vi "CPP-BLplotter.vi"(0 "Plot Array":cluster{dbl[], dbl[]}[](array[cluster])=[{[500.0, 500.0, 953.54, 215.0, 270.0, 320.0, 445.0, 525.0, 600.0, 675.0, 750.0, 825.0, 900.0, 960.0, 1010.0, 1060.0], [4.614524, 4.54365, 5.818368, 0.1374656, 0.6662545, 1.465458, 3.619824, 4.848976, 5.887329, 5.940571, 6.152151, 5.717487, 5.600293, 5.40069, 5.154843, 5.121789]}, {[100.0, 150.0, 215.0, 270.0, 320.0, 445.0, 525.0, 600.0, 675.0, 750.0, 825.0, 900.0, 960.0, 1010.0, 1060.0], [0.002314715, -0.00693192, 0.120417, 0.6880509, 1.519176, 3.513709, 5.065183, 6.116033, 6.096773, 5.938465, 5.593788, 5.5597, 5.387002, 5.304077, 4.887903]}] {"?" format="%.2f"; "?" format="%.2f"}, 1 "Job Directory":path=path "/G4_2_HD/Users/paulhayden/Documents/Projects/Westlakes_resolution") -> (2 "Saved Automatically?":bool, 3 "gnuplotScript":string="set term epslatex\nset output \"Plot.eps\"\nset xlabel '$Distance~(m)$'\nset ylabel '$DF~(s/m^3)\\times10^6$'\nset samples 1000\nset pointsize 1.00\nset title '$B38~Centreline~Glc$' 0, 0\nset size 0.75,0.9\n\n#set key 450, -2.5833\n unset key\nset label 1 '~~~~~~~~~~~Angle~(deg)~=~0' at -100, -2.58\nset label 2 '~~~~~~~~~~~Height~(m)~=~5' at -100, -3.27\n set xrange [0 : 500] \n# set autoscale x \n set yrange [0.10000 : 7]\n# set autoscale y \n\nplot \"B38_Centreline_Glc.dat\" index 0 using 1:2 axes x1y1 title '$File=B38R~DDD.xls$' with points 1 1, \\\n\"B38_Centreline_Glc.dat\" index 1 using 1:2 axes x1y1 title '$File=B38R~DDD~1.xls$' with points 1 3", 4 "Plot data file":path)   [LabVIEW 2013]
uses:
  Results_plotter_Global.vi
panel:
  in  "Tab Control":enum32{"Good Shit", "Boring Shit"}(tab)
  in  "HeightJitterFraction":dbl=0.03
  in  "Spectra Files:":path
  out "Spectrum":cluster{dbl[], dbl[]}[](graph)
  in  "Cancel Button":bool
  in  "Print Button":bool
  out "U,L(U)":cluster{dbl[], dbl[]}[](graph)
  out "TI,Sigma":cluster{dbl[], dbl[]}[](graph)
  in  "Use for:":enum16{"\nU", "\nLambda", "\nTI", "\nSigma"}[](array[ring])=[enum."\nU", enum."\nTI", enum."\nSigma", enum."\nLambda"]
  out "Incoming Titles":string[](array[string])
  in  "Plot Title":u16(ring) items=["Title String Only", "Number of Measurements", "Date::", "Profile::", "Multi Run:Start Time:", "Multi Run:Row:Type", "Multi Run:Row:Number", "Point:Time:", "Time:Stamp:", "Measuring:Instrument:Type", "Comments::", "Run:Messages:", "X_{HF}:(mm):", "Y_{HF}:(mm):", "Z_{HF}:(mm):", "X_{5HP}:(mm):", "Y_{5HP}:(mm):", "Z_{5HP}:(mm):", "Repeat::", "U_{HF}/U_{ref}::", "U_{5HP}/U_{ref}::", "U_{HF}/U_{5HP}::", "TI_{HF}:%:", "\\sigma_{HF}/U_{ref}::", "TI_{U(5HP)}:%:", "Vmag_{5HP}/U_{ref}::", "V_{5HP}/U_{5HP}::", "W_{5HP}/U_{5HP}::", "U_{ref}::", "U_{HF}::", "L(U):Est:(m)", "Tau(HF)::", "uhf^2::", "uhf^3/(uhf^2)^1.5::", "(uhf^4/(uhf^2)^2) -3::", "HW (Uhf):Standard Error:in Mean", "HW (Uhf):Standard Error:in Variance", "HW:Cal:", "Vmag_{5HP}::", "U_{5HP}::", "V_{5HP}::", "W_{5HP}::", "Vmag_SD::", "U_SD::", "V_SD::", "W_SD::", "Tau(5HP1)::(nose)", "Tau(5HP2)::(bottom)", "Tau(5HP3)::(top)", "Tau(5HP4)::(side)", "Tau(5HP5)::(side)", "GoodFraction::", "5HP:Mode:", "5HP:ReturnType:", "Reference:Temperature:Used for Corrections", "Atmos:Pressure:Used for Corrections", "Av Analogue:Sampling:Rate", "No of:Analogue:Samples", "No Of:Measurement:Blocks", "Flow:Measurement:Time", "X:(URef):(mm)", "Y:(URef):(mm)", "Z:(URef):(mm)", "Original:Results:Filename", "Current:Data:Filename", "Current:Data File:1st Folder level", "Current:Data File:2nd Folder level", "Current:Data File:3rd Folder level", "Current:Data File:4th Folder level", "Current:File:Number", "Raw:Data:Filename"]
  in  "Filename Max length":i32=255
  out "Final Title":string="B38 Centreline Glc"
  out "Path":path
  in  "Plot Title Post Block":string
  in  "Plot Title Pre Block":string
  in  "Show Script Editor?":bool
  out "t":string
  in  "OpenLogfile?":bool
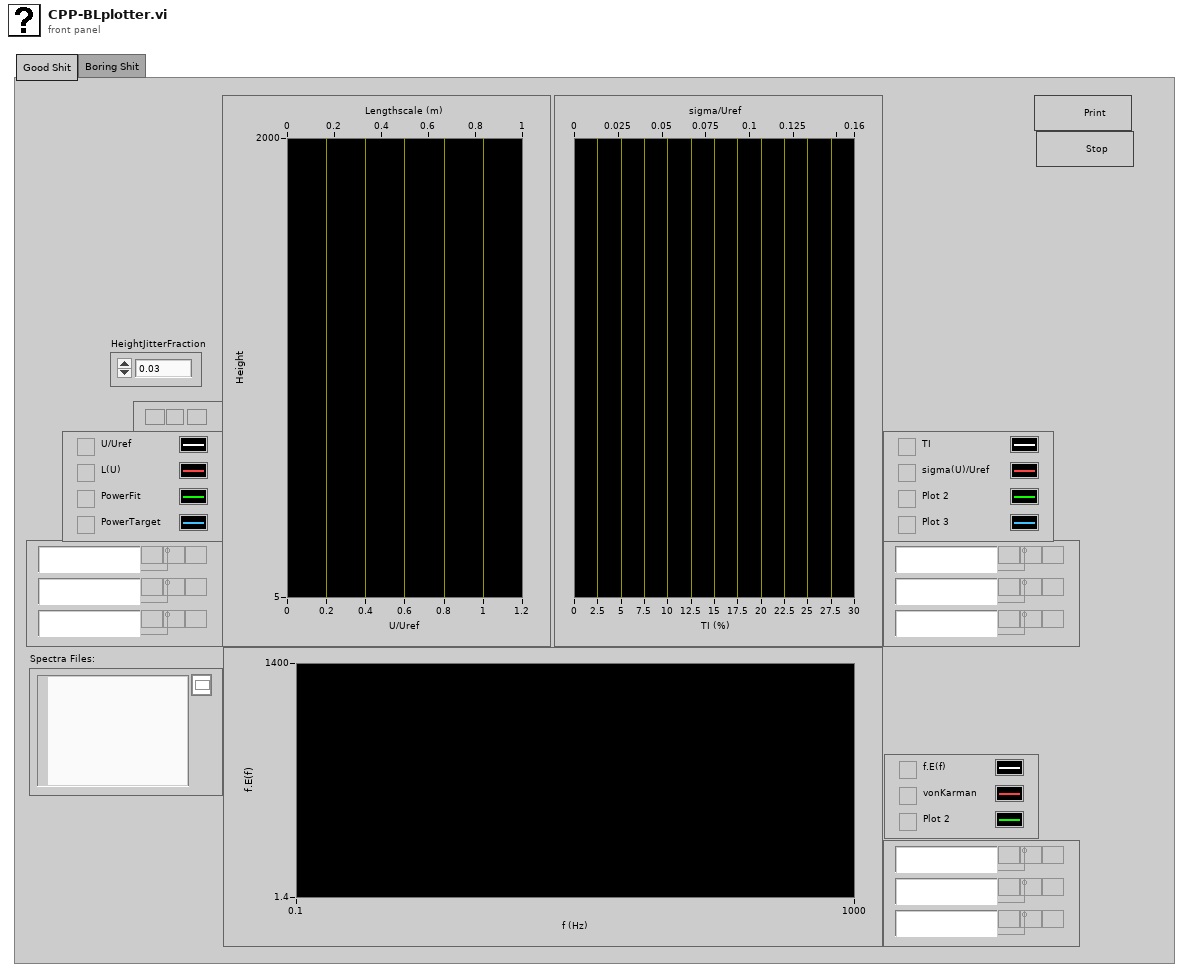
[diagram p1: front panel]
types:
  T1 = typedef "LVRangeTypeDef.ctl" = cluster{"Minimum":dbl, "Maximum":dbl, "Increment":dbl, "Minor Increment":dbl, "Start":dbl}
  T2 = typedef "minAndMax.ctl" = cluster{"Min":T3, "Max":T3}
  T3 = typedef "AutoManualNumber.ctl" = cluster{"Auto":bool, "Value":dbl}
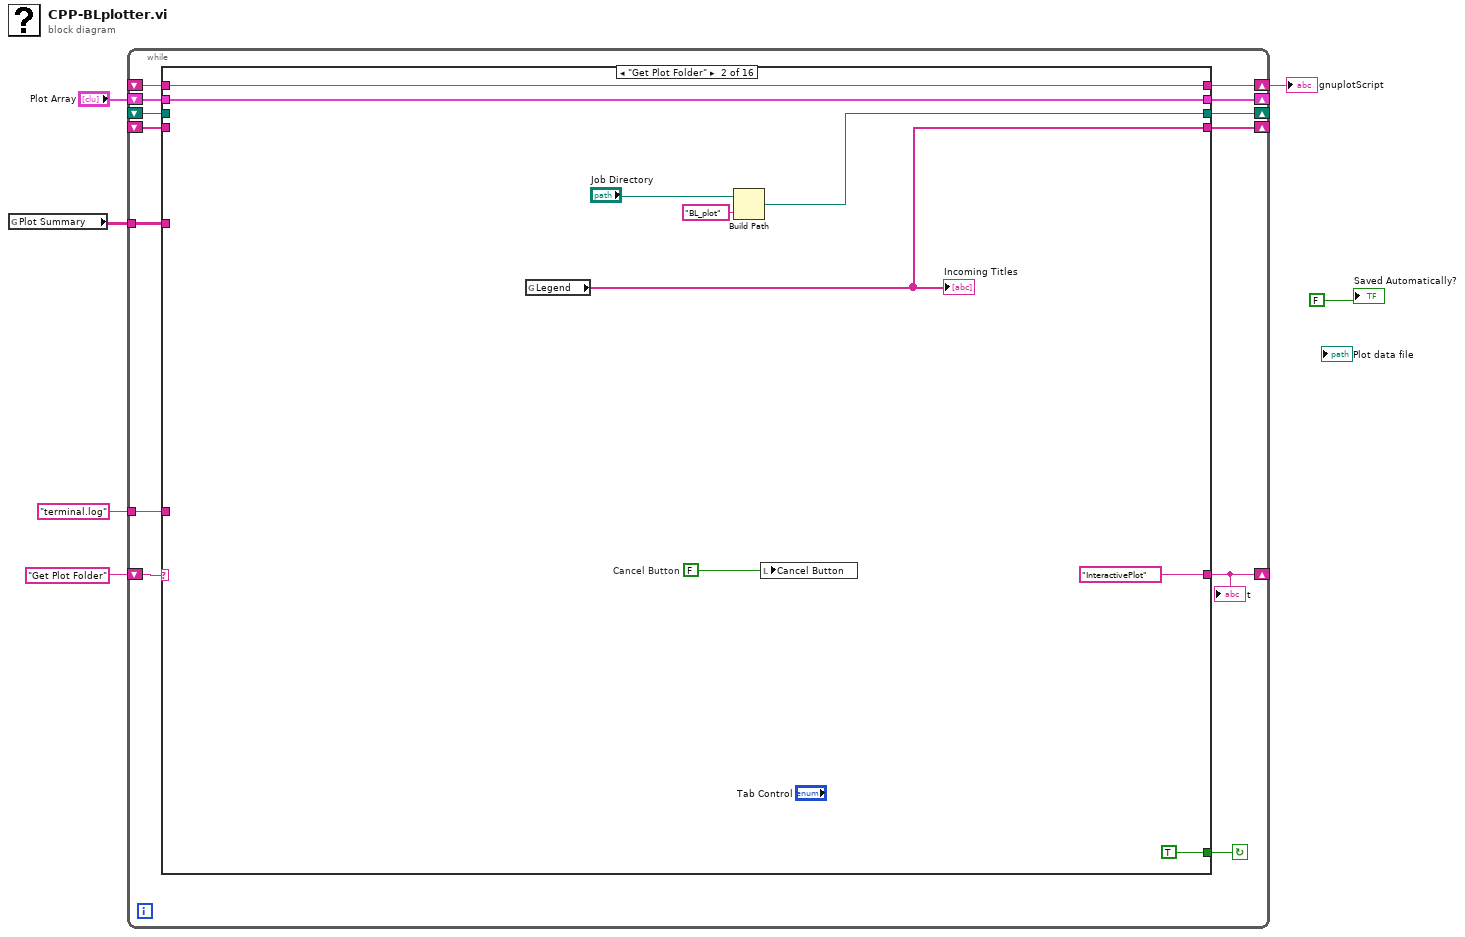
[diagram p0: block diagram]
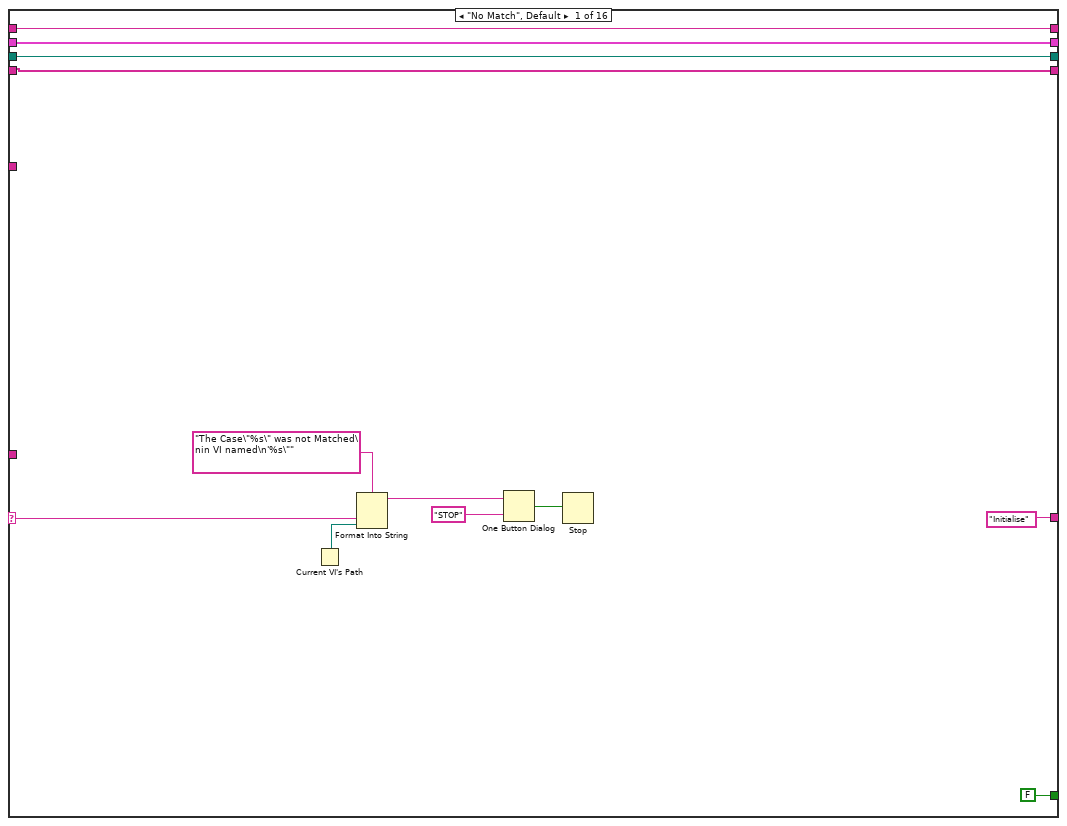
[diagram p2: hidden frame]
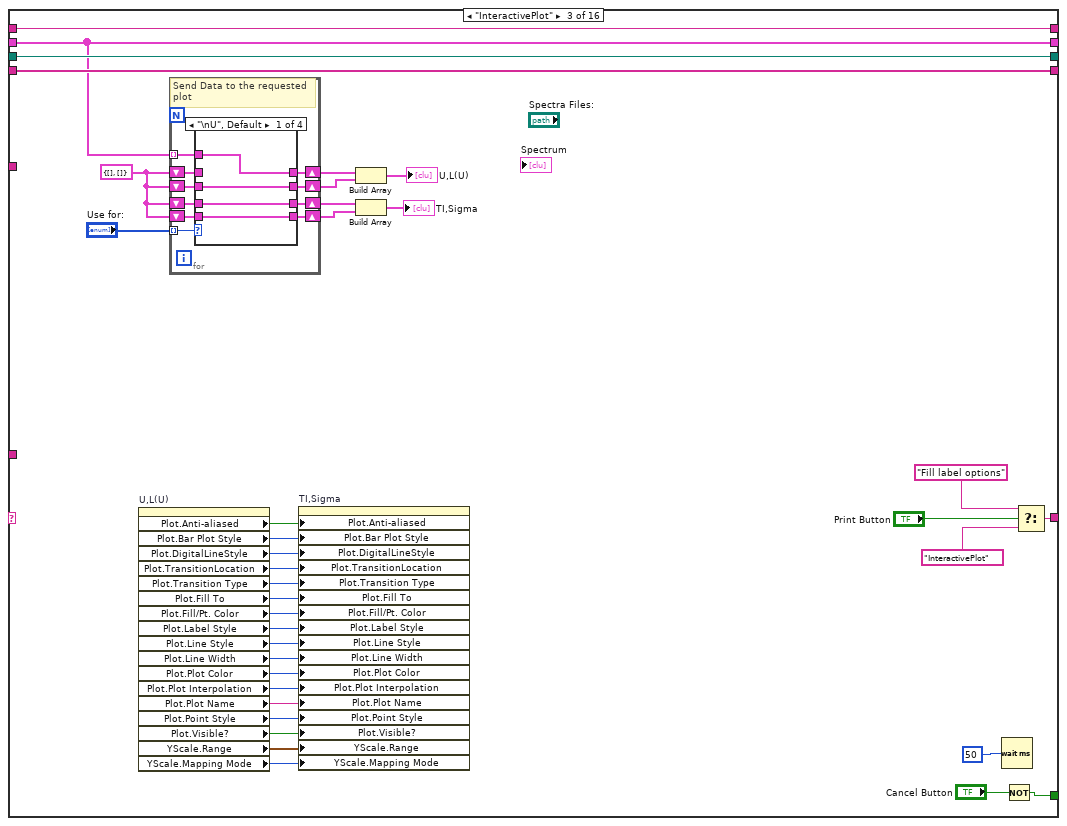
[diagram p3: hidden frame]
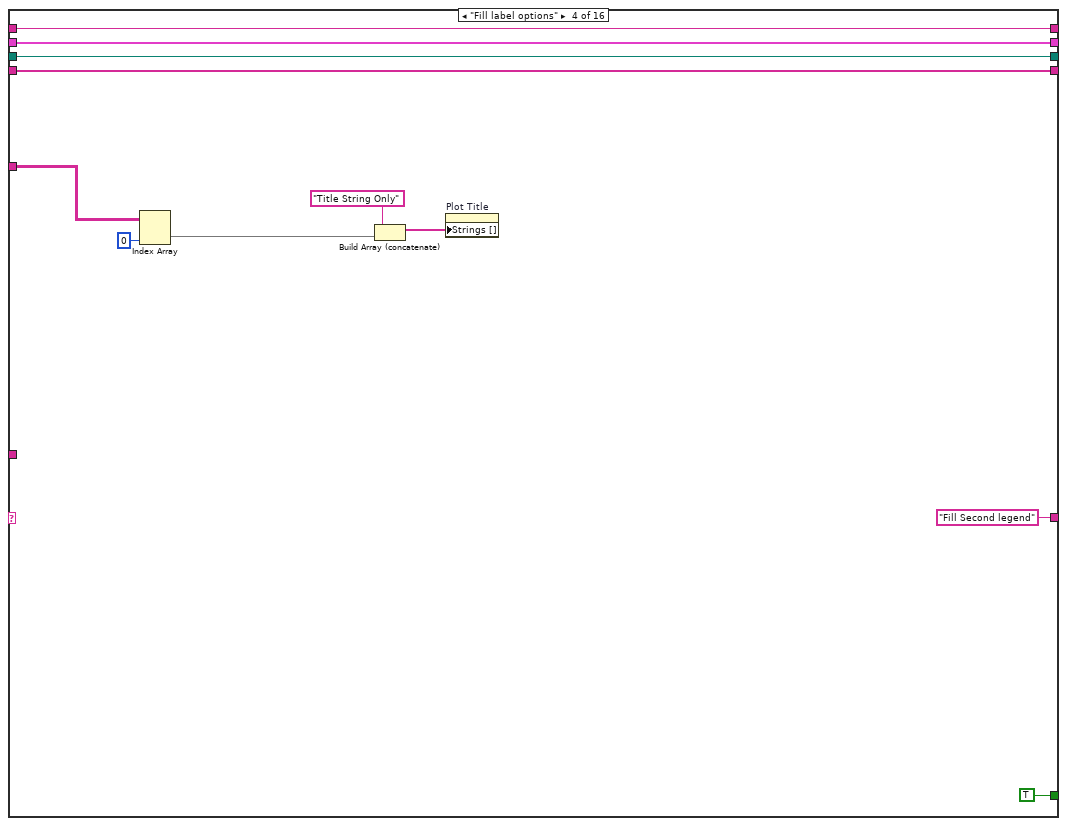
[diagram p7: hidden frame]
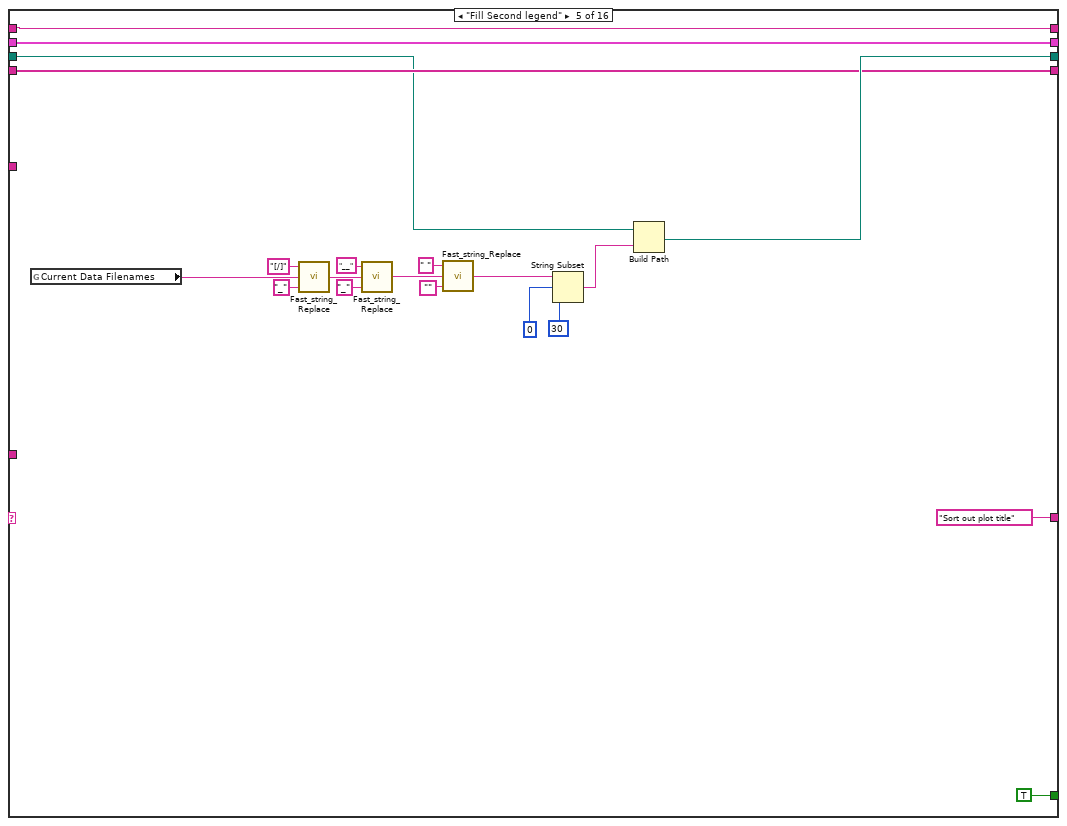
[diagram p8: hidden frame]
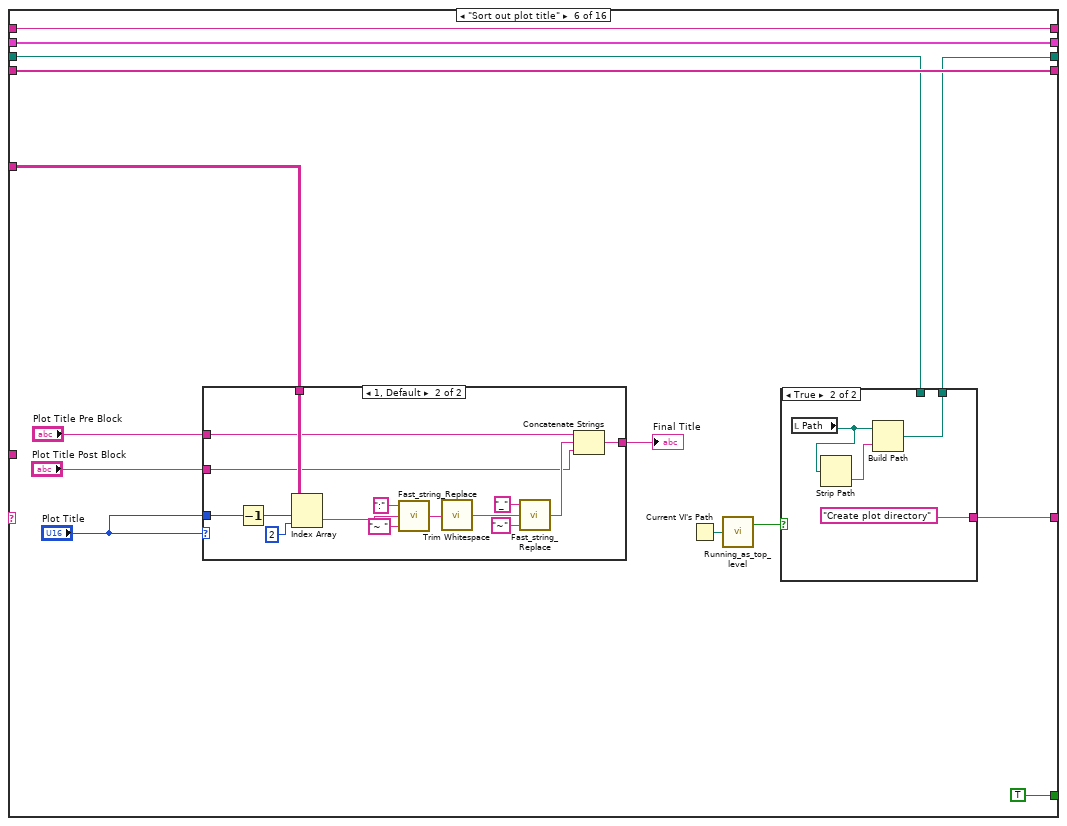
[diagram p9: hidden frame]
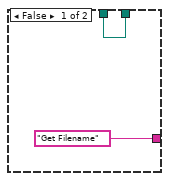
[diagram p10: hidden frame]
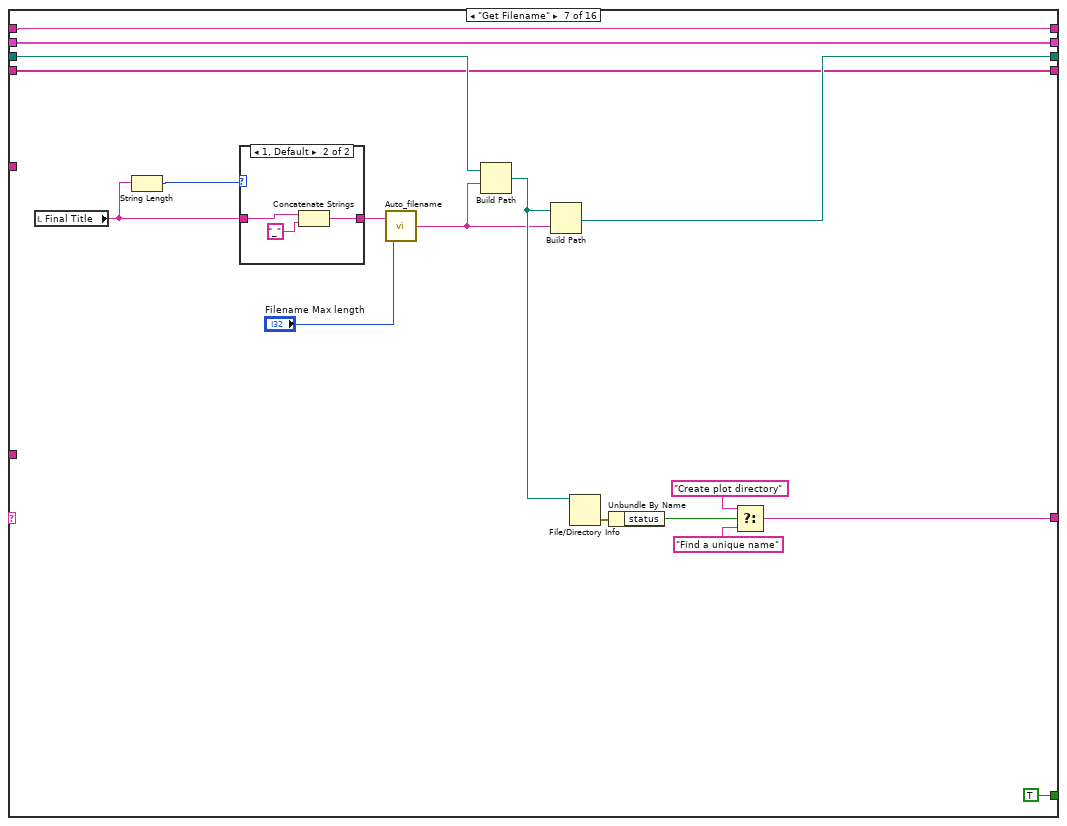
[diagram p12: hidden frame]
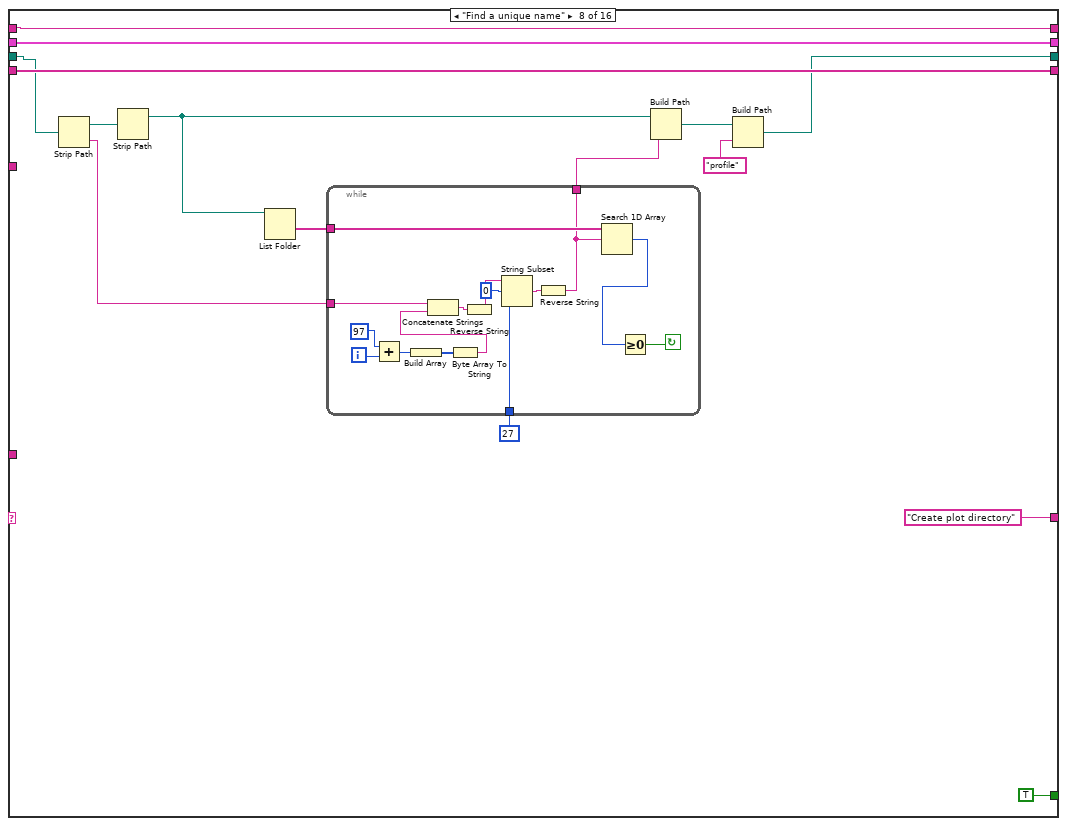
[diagram p14: hidden frame]
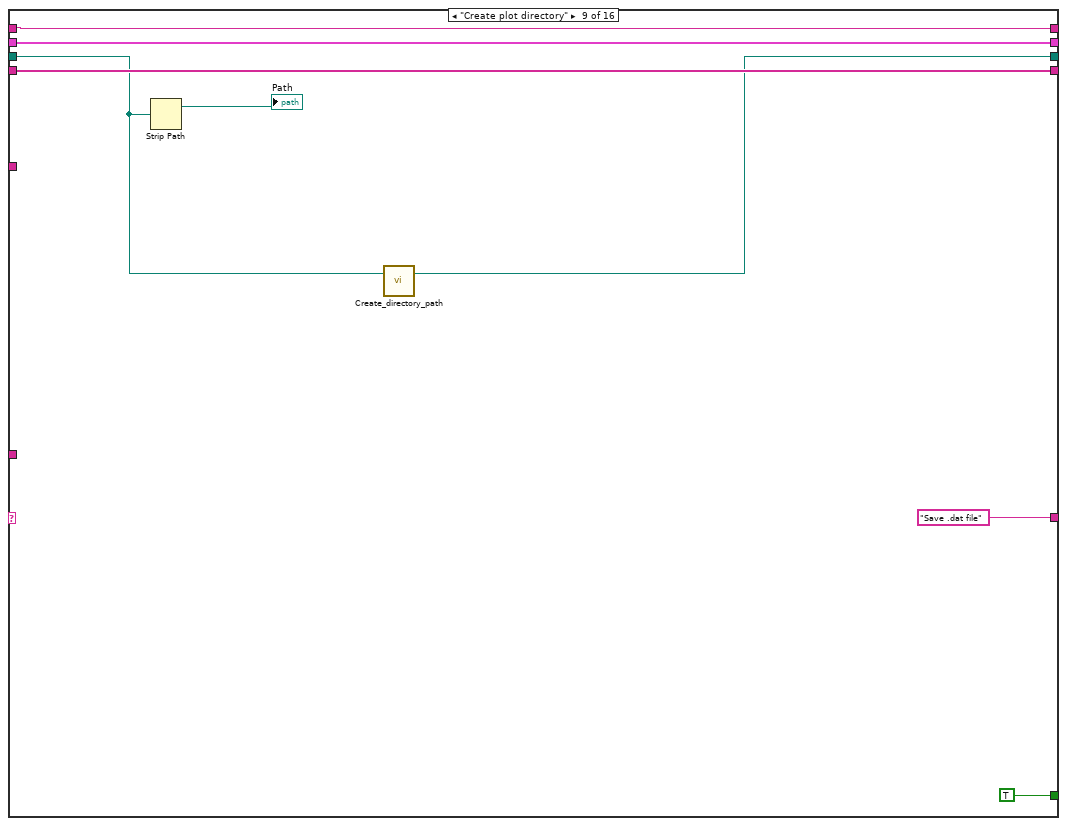
[diagram p15: hidden frame]
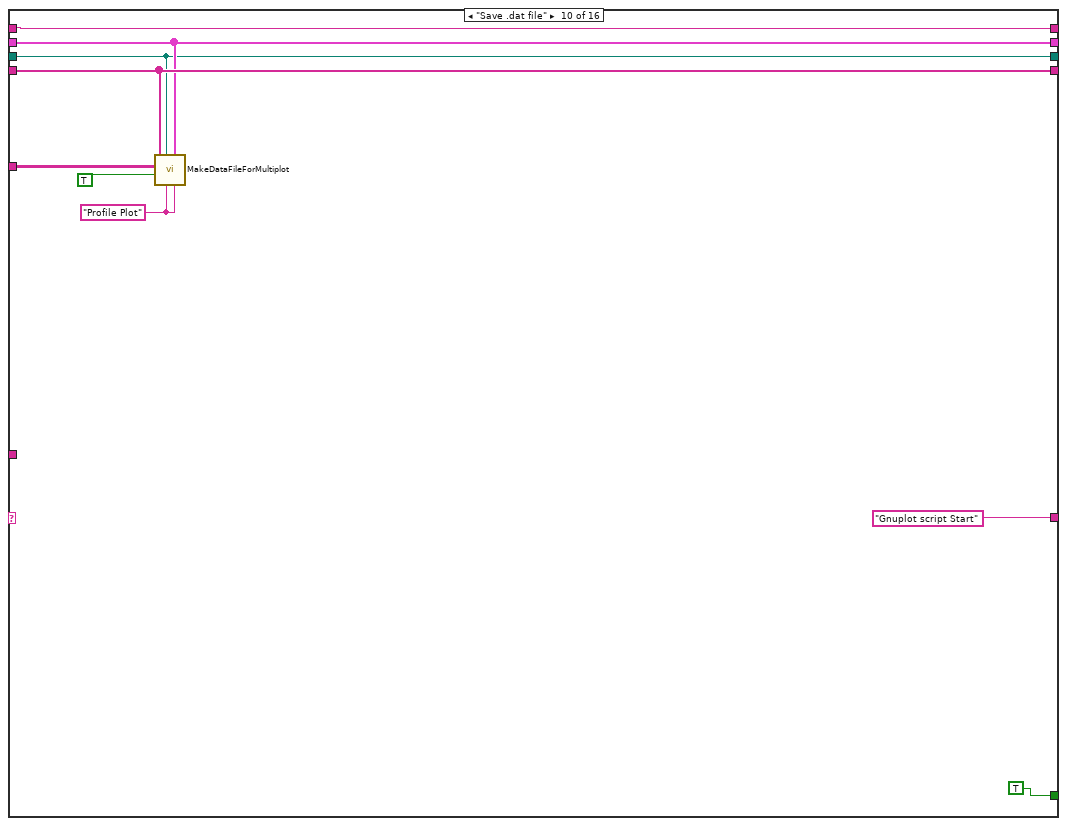
[diagram p16: hidden frame]
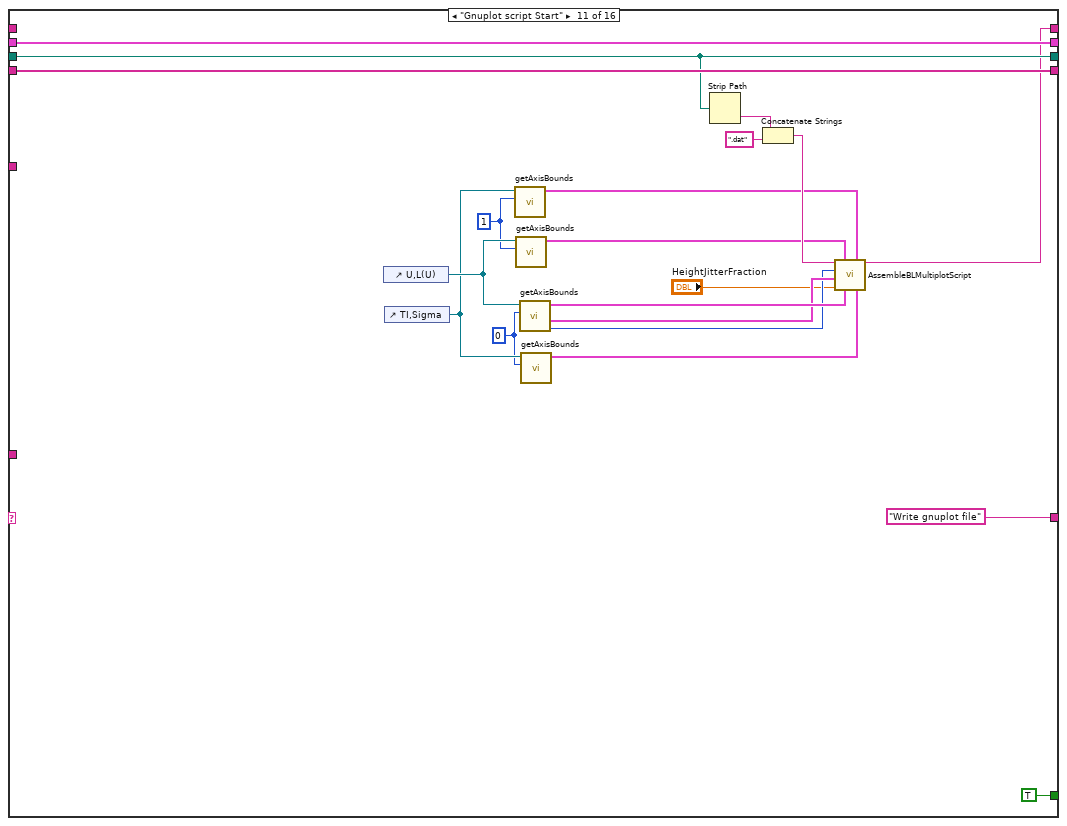
[diagram p17: hidden frame]
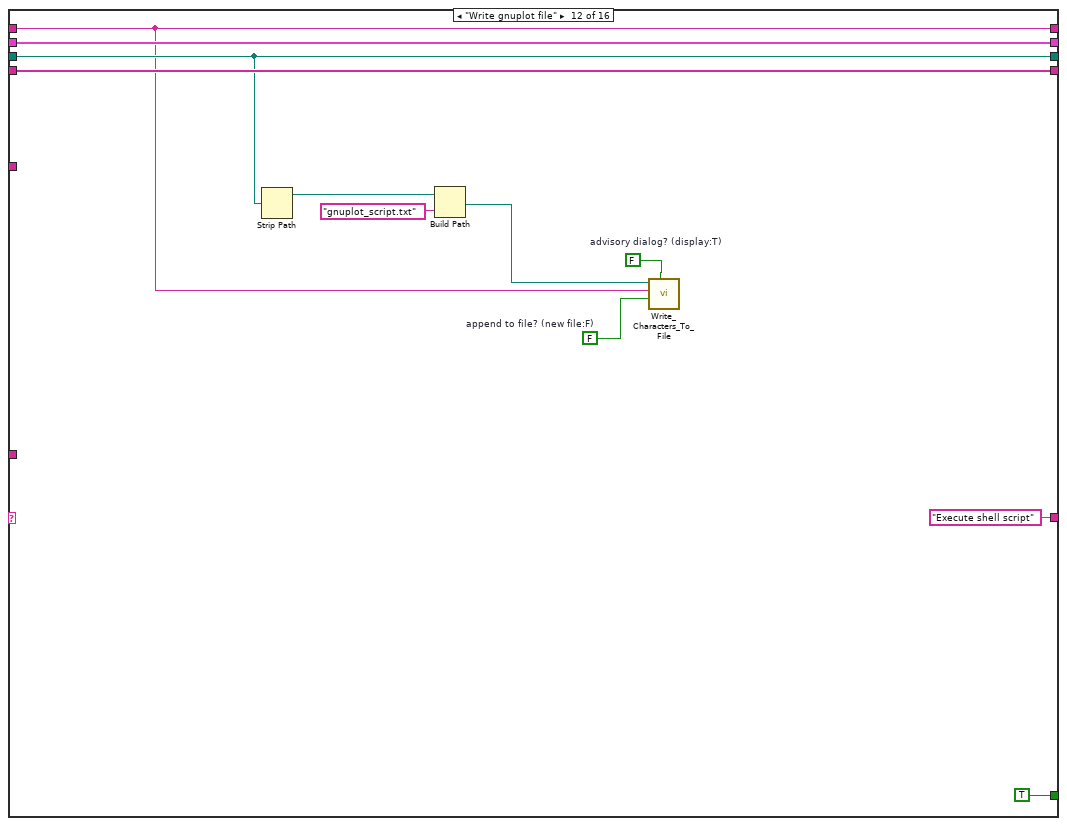
[diagram p18: hidden frame]
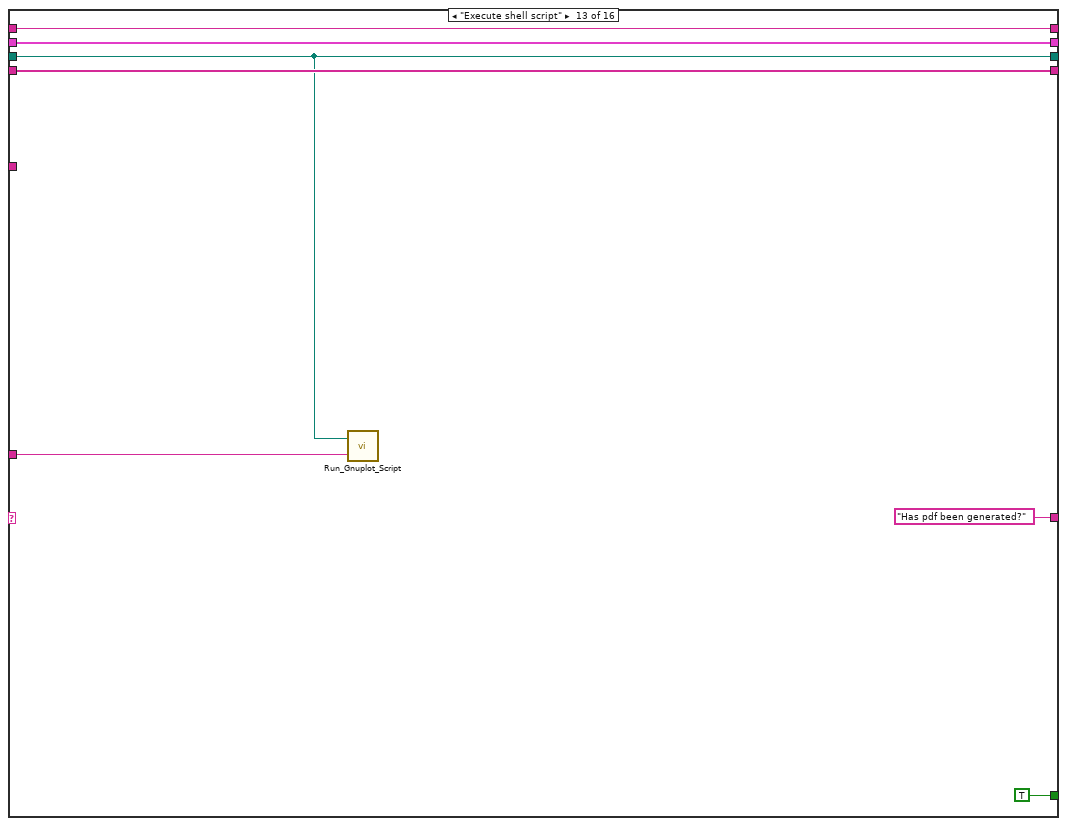
[diagram p19: hidden frame]
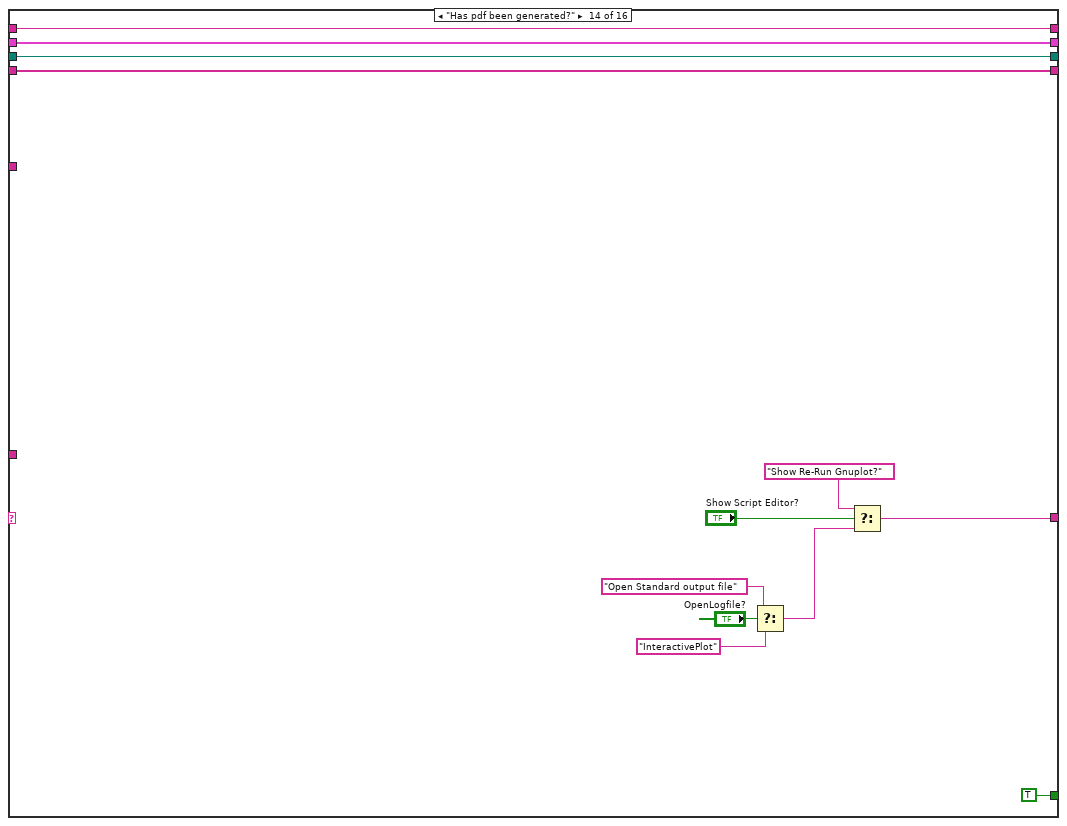
[diagram p20: hidden frame]
diagram:
  n1 = global read "Results_plotter_Global.vi" "Plot Summary"() -> (w5:string[][])
  n2 = while {
    shift-left: "Get Plot Folder" -> [w18]
    shift-right: [w7] -> _
    tunnel: w5 -> [w17]
    shift-right: [w16] -> _
    shift-left: _ -> [w15]
    shift-right: [w13] -> _
    shift-left: "Plot Array" -> [w14]
    shift-right: [w11] -> w4
    shift-left: _ -> [w12]
    shift-right: [w10] -> _
    shift-left: _ -> [w9]
    tunnel: "terminal.log" -> [w8]
    stop <- w19 continue-if-true
    n3 = case shown="\"Get Plot Folder\"" w18 {
      selector: w18 -> [w20 _ _ _ _ _ _ _ _ _ _ _ _ _ _ _]
      tunnel: [FALSE TRUE w68 TRUE ("Top Level") TRUE ("Top Level") TRUE ("Top Level") TRUE ("Top Level") TRUE ("Top Level") TRUE TRUE ("Top Level") TRUE ("Top Level") TRUE ("Top Level") TRUE ("Top Level") TRUE ("Top Level") TRUE ("Top Level") TRUE ("Top Level")] -> w19
      tunnel: ["Initialise" "InteractivePlot" w73 "Fill Second legend" "Sort out plot title" w135 w184 "Create plot directory" "Save .dat file" "Gnuplot script Start" "Write gnuplot file" ("t") "Execute shell script" ("t") "Has pdf been generated?" ("t") w280 "End" "InteractivePlot" ("t")] -> w7
      tunnel: w17 -> [_ _ _ w113 _ w142 _ _ _ w234 _ _ _ _ _ _]
      tunnel: [w24 w37 w76 w107 w133 w137 w185 w192 w225 w231 w254 w262 w270 w284 w289 w299] -> w16
      tunnel: w15 -> [w24 _ w76 w107 w129 w136 w181 w199 w224 w231 w254 w262 w270 w284 w289 w299]
      tunnel: w14 -> [w23 w34 w45 w108 w132 w147 w183 w202 w228 w232 w257 w268 w275 w287 w294 w304]
      tunnel: [w23 w34 w45 w108 w132 w147 w183 w202 w228 w232 w257 w268 w275 w287 w294 w304] -> w13
      tunnel: w12 -> [w22 w36 w74 w109 w131 w143 w182 w201 w227 w237 _ w258 w273 w285 w292 w302]
      tunnel: [w22 w36 w74 w109 w131 w143 w182 w201 w227 w237 w251 w258 w273 w285 w292 w302] -> w11
      tunnel: [w21 w32 w75 w106 w130 w146 w180 w200 w226 w233 w256 w263 w274 w286 w293 w303] -> w10
      tunnel: w9 -> [w21 _ w75 w106 w130 w146 w180 w200 w226 w233 w256 w263 w274 w286 w293 w303]
      tunnel: w8 -> [_ _ _ _ _ _ _ _ _ _ _ _ w269 _ _ w297]
      frame "No Match", Default {
        n4 = Current VI's Path() -> (path=w26:path)
        n5 = Format Into String(format string="The Case\"%s\" was not Matched\nin VI named\n'%s\"" ("Format String"), w20, w26) -> (resulting string=w29:string)  [unwired: 2 in, 1 out]
        n6 = One Button Dialog(message=w29, button name ("OK")="STOP") -> (true=w27:bool)
        n7 = Stop(stop? (T)=w27) -> ()
      }
      frame "Get Plot Folder" {
        w33 = FALSE  # Cancel Button
        n8 = global read "Results_plotter_Global.vi" "Legend"() -> (w32:string[])
        "Incoming Titles" <- w32
        n9 = Build Path(base path="Job Directory", name or relative path="BL_plot") -> (appended path=w37:path)
        n10 = local write "Cancel Button"(w33) -> ()
      }
      frame "InteractivePlot" {
        w44 = cluster{dbl[], dbl[]} {[], []}
        n11 = property on="U,L(U)" class="XYGraph (strict)"() -> ("Plot.Anti-aliased"=w50:bool, "Plot.Bar Plot Style"=w51:u8, "Plot.DigitalLineStyle"=w52:u8, "Plot.TransitionLocation"=w53:u8, "Plot.Transition Type"=w54:u8, "Plot.Fill To"=w55:i16, "Plot.Fill/Pt. Color"=w56:u32, "Plot.Label Style"=w57:u8, "Plot.Line Style"=w58:u8, "Plot.Line Width"=w59:u8, "Plot.Plot Color"=w60:u32, "Plot.Plot Interpolation"=w61:u8, "Plot.Plot Name"=w62:string, "Plot.Point Style"=w63:u8, "Plot.Visible?"=w64:bool, "YScale.Range"=w65:T1, "YScale.Mapping Mode"=w66:u8)  [unwired: 2 in, 2 out]
        n12 = for {
          tunnel: "Use for:" -> [w81] mode=indexing
          shift-right: [w86] -> w49
          shift-left: w44 -> [w80]
          shift-right: [w83] -> w47
          shift-left: w44 -> [w79]
          shift-right: [w82] -> w46
          shift-left: w44 -> [w78]
          shift-right: [w84] -> w48
          shift-left: w44 -> [w85]
          tunnel: w45 -> [w77] mode=indexing
          # "Send Data to the requested plot"
          n13 = case shown="\"\\nU\", Default" w81 {
            tunnel: [w90 w92 w96 w101] -> w86
            tunnel: w85 -> [_ w91 w97 w102]
            tunnel: [w87 w91 w97 w102] -> w84
            tunnel: [w89 w94 w98 w100] -> w83
            tunnel: [w88 w93 w95 w99] -> w82
            tunnel: w80 -> [w90 _ w96 w101]
            tunnel: w79 -> [w89 w94 _ w100]
            tunnel: w78 -> [w88 w93 w95 _]
            tunnel: w77 -> [w87 w92 w98 w99]
            frame "\nU", Default {
            }
            frame "\nLambda" {
            }
            frame "\nTI" {
            }
            frame "\nSigma" {
            }
          }
        }
        n14 = property on="TI,Sigma" class="XYGraph (strict)"("Plot.Anti-aliased"=w50, "Plot.Bar Plot Style"=w51, "Plot.DigitalLineStyle"=w52, "Plot.TransitionLocation"=w53, "Plot.Transition Type"=w54, "Plot.Fill To"=w55, "Plot.Fill/Pt. Color"=w56, "Plot.Label Style"=w57, "Plot.Line Style"=w58, "Plot.Line Width"=w59, "Plot.Plot Color"=w60, "Plot.Plot Interpolation"=w61, "Plot.Plot Name"=w62, "Plot.Point Style"=w63, "Plot.Visible?"=w64, "YScale.Range"=w65, "YScale.Mapping Mode"=w66) -> ()  [unwired: 2 in, 2 out]
        n15 = Build Array(w48, w49) -> (→"U,L(U)":cluster{dbl[], dbl[]}[])
        n16 = Build Array(w47, w46) -> (→"TI,Sigma":cluster{dbl[], dbl[]}[])
        n17 = Wait (ms)(milliseconds to wait=u32 50) -> ()  [unwired: 1 out]
        n18 = Not(x="Cancel Button") -> (.not. x?=w68:bool)
        n19 = Select(t="Fill label options", s="Print Button", f="InteractivePlot") -> (s? t:f=w73:string)
      }
      frame "Fill label options" {
        n20 = Index Array(array=w113, index (col)=0 ("disabled index (col)")) -> (element=w104:string[])  [unwired: 1 in]
        n21 = Build Array (concatenate)("Title String Only", w104) -> (w103:string[])
        n22 = property on="Plot Title" class="Ring (strict)"("Strings []"=w103) -> ()  [unwired: 2 in, 2 out]
      }
      frame "Fill Second legend" {
        n23 = global read "Results_plotter_Global.vi" "Current Data Filenames"() -> (w118:string)
        n24 = call "Fast_string_Replace.vi"("Replace match with:"="_", "Input String"=w118, "regular expression"="[/]") -> ("Output String"=w122:string)  [unwired: 2 out]
        n25 = call "Fast_string_Replace.vi"("Replace match with:"="_", "Input String"=w122, "regular expression"="__") -> ("Output String"=w119:string)  [unwired: 2 out]
        n26 = call "Fast_string_Replace.vi"("Replace match with:"="", "Input String"=w119, "regular expression"=" ") -> ("Output String"=w117:string)  [unwired: 2 out]
        n27 = String Subset(string=w117, offset (0)=0, length (rest)=30 ("length (rest)")) -> (substring=w116:string)
        n28 = Build Path(base path=w129, name or relative path=w116) -> (appended path=w133:path)
      }
      frame "Sort out plot title" {
        n29 = case shown="1, Default" "Plot Title" {
          tunnel: [w154 w159] -> w141
          tunnel: "Plot Title Pre Block" -> [w154 w158]
          tunnel: w142 -> [_ w162]
          tunnel: "Plot Title" -> [_ w161]
          tunnel: "Plot Title Post Block" -> [_ w155]
          frame 0 {
          }
          frame 1, Default {
            n30 = Decrement(x=w161) -> (x-1=w160:u16)
            n31 = Index Array(array=w162, index (row)=w160, index (col)=u16 2 ("y")) -> (element=w165:string)
            n32 = call "Fast_string_Replace.vi"("Replace match with:"="~ ", "Input String"=w165, "regular expression"=":") -> ("Output String"=w164:string)  [unwired: 2 out]
            n33 = call <vilib>:"Trim Whitespace.vi"("string"=w164) -> ("trimmed string"=w163:string)  [unwired: 1 in]
            n34 = call "Fast_string_Replace.vi"("Replace match with:"="~", "Input String"=w163, "regular expression"="_") -> ("Output String"=w157:string)  [unwired: 2 out]
            n35 = Concatenate Strings(w158, w157, w155) -> (w159:string)
          }
        }
        "Final Title" <- w141
        n36 = Current VI's Path() -> (path=w140:path)
        n37 = call "Running_as_top_level.vi"("Vi path name"=w140) -> ("Top Level"=w138:bool)  [unwired: 1 out]
        n38 = case shown="True" w138 {
          tunnel: [w149 w152] -> w137
          tunnel: w136 -> [w149 _]
          tunnel: ["Get Filename" ("t") "Create plot directory"] -> w135
          frame False {
          }
          frame True {
            n39 = local read "Path"() -> (w151:path)
            n40 = Strip Path(path=w151) -> (name=w150:string)  [unwired: 1 out]
            n41 = Build Path(base path=w151, name or relative path=w150) -> (appended path=w152:path)
          }
        }
      }
      frame "Get Filename" {
        n42 = local read "Final Title"() -> (w170:string)
        n43 = String Length(string=w170) -> (length=w172:i32)
        n44 = case shown="1, Default" w172 {
          tunnel: [w187 w188] -> w171
          tunnel: w170 -> [w187 w190]
          frame 0 {
          }
          frame 1, Default {
            n45 = Concatenate Strings(w190, "_") -> (w188:string)
          }
        }
        n46 = call "Auto_filename.vi"("Filename Max length"="Filename Max length", "Prefix"=w171) -> ("Filename"=w174:string)
        n47 = Build Path(base path=w181, name or relative path=w174) -> (appended path=w178:path)
        n48 = Build Path(base path=w178, name or relative path=w174) -> (appended path=w185:path)
        n49 = File/Directory Info(path=w178) -> (error out=w179:errorcluster)  [unwired: 1 in, 6 out]
        n50 = Unbundle By Name(w179) -> ("status"=w177:bool)
        n51 = Select(t="Create plot directory", s=w177, f="Find a unique name") -> (s? t:f=w184:string)
      }
      frame "Find a unique name" {
        n52 = Strip Path(path=w199) -> (stripped path=w198:path, name=w197:string)
        n53 = Strip Path(path=w198) -> (stripped path=w195:path)  [unwired: 1 out]
        n54 = List Folder(path=w195) -> (folder names=w196:string[])  [unwired: 1 in, 5 out]
        n55 = while {
          tunnel: w197 -> [w220]
          tunnel: 27 ("Max Length") -> [w219]
          tunnel: [w208] -> w194
          tunnel: w196 -> [w209]
          i -> [w210]
          stop <- w206 continue-if-true
          n56 = Add(x=97, y=w210) -> (x+y=w217:i32)
          n57 = Build Array(w217) -> (w218:i32[])
          n58 = Byte Array To String(unsigned byte array=w218) -> (string=w215:string)
          n59 = Concatenate Strings(w220, w215) -> (w213:string)
          n60 = Reverse String(1:w213) -> (0:w214:string)
          n61 = String Subset(string=w214, offset (0)=0, length (rest)=w219) -> (substring=w212:string)
          n62 = Reverse String(1:w212) -> (0:w208:string)
          n63 = Search 1D Array(1D array=w209, element=w208) -> (index of element=w207:i32)  [unwired: 1 out]
          n64 = Greater Or Equal To 0?(x=w207) -> (x >= 0?=w206:bool)
        }
        n65 = Build Path(base path=w195, name or relative path=w194) -> (appended path=w193:path)
        n66 = Build Path(base path=w193, name or relative path="profile") -> (appended path=w192:path)
      }
      frame "Create plot directory" {
        n67 = Strip Path(path=w224) -> (stripped path=→"Path":path)  [unwired: 1 out]
        n68 = call "Create_directory_path.vi"("Path name"=w224) -> ("Path name Out"=w225:path)  [unwired: 1 in, 1 out]
      }
      frame "Save .dat file" {
        w229 = "Profile Plot" ("X Axis Name")
        n69 = call "MakeDataFileForMultiplot.vi"("Y Axis Name"=w229, "Plot Array"=w232, "X Axis Name"=w229, "Path"=w231, "Transpose"=TRUE, "Plot Summary"=w234, "Legend"=w233) -> ()  [unwired: 5 in]
      }
      frame "Gnuplot script Start" {
        w245 = 1 ("Active X Scale")
        w246 = 0 ("Active X Scale")
        n70 = control-ref of="U,L(U)"() -> (w248:refnum<vi>)
        n71 = control-ref of="TI,Sigma"() -> (w247:refnum<vi>)
        n72 = call "getAxisBounds.vi"("Active X Scale"=w245, "XYGraph in"=w247) -> ("Xbounds"=w244:T2)  [unwired: 6 in, 3 out]
        n73 = call "getAxisBounds.vi"("Active X Scale"=w245, "XYGraph in"=w248) -> ("Xbounds"=w243:T2)  [unwired: 6 in, 3 out]
        n74 = call "getAxisBounds.vi"("Active X Scale"=w246, "XYGraph in"=w248) -> ("YMapping"=w239:enum8{"Lin", "Log"}, "Ybounds"=w240:T2, "Xbounds"=w242:T2)  [unwired: 6 in, 1 out]
        n75 = call "getAxisBounds.vi"("Active X Scale"=w246, "XYGraph in"=w247) -> ("Xbounds"=w241:T2)  [unwired: 6 in, 3 out]
        n76 = Strip Path(path=w254) -> (name=w252:string)  [unwired: 1 out]
        n77 = Concatenate Strings(w252, ".dat" ("string")) -> (w250:string)
        n78 = call "AssembleBLMultiplotScript.vi"("ProfileFilename"=w250, "lambdaBounds"=w243, "sigma/U bounds"=w244, "Mapping"=w239, "HeightAxisBounds"=w240, "jitterFraction"="HeightJitterFraction", "U/UrefBounds"=w242, "TI bounds"=w241) -> ("gnuplotOut"=w251:string)  [unwired: 7 in]
      }
      frame "Write gnuplot file" {
        w265 = FALSE  # append to file? (new file:F)
        w266 = FALSE  # advisory dialog? (display:T)
        n79 = Strip Path(path=w262) -> (stripped path=w259:path)  [unwired: 1 out]
        n80 = Build Path(base path=w259, name or relative path="gnuplot_script.txt") -> (appended path=w267:path)
        n81 = call "Write_Characters_To_File.vi"("file path (dialog if empty)"=w267, "advisory dialog? (display:T)"=w266, "character string"=w258, "append to file? (new file:F)"=w265) -> ()  [unwired: 1 in, 4 out]
      }
      frame "Execute shell script" {
        n82 = call "Run_Gnuplot_Script.vi"("logfileName"=w269, "workingDirectory"=w270) -> ()
      }
      frame "Has pdf been generated?" {
        n83 = Select(t="Open Standard output file" ("f"), s="OpenLogfile?", f="InteractivePlot" ("t")) -> (s? t:f=w277:string)
        n84 = Select(t="Show Re-Run Gnuplot?", s="Show Script Editor?", f=w277) -> (s? t:f=w280:string)
      }
      frame "Show Re-Run Gnuplot?" {
        (unwired) "InteractivePlot" ("t")
        n85 = Strip Path(path=w289) -> (stripped path=w288:path)  [unwired: 1 out]
        n86 = call "Re_run_Gnuplot.vi"("Plot folder (dialog if empty)"=w288) -> ()  [unwired: 4 out]
      }
      frame "Open Standard output file" {
        n87 = Strip Path(path=w299) -> (stripped path=w296:path)  [unwired: 1 out]
        n88 = Format Into String(format string="open \"%s\"", w297) -> (resulting string=w295:string)  [unwired: 2 in, 1 out]
        n89 = call <vilib>:"System Exec.vi"("working directory"=w296, "command line"=w295) -> ()  [unwired: 4 in, 6 out]
      }
    }
    "t" <- w7
  }
  "gnuplotScript" <- w4
  "Saved Automatically?" <- FALSE
